vi "ConvertEventListToTriggerEvents.vi"(11 "Event List":string) -> (3 "Trigger Events":enum16{"Source", "Delay", "Sense", "None"}[](array[ring]))   [LabVIEW 2014, in "Keithley-6482-Visa.lvlib"]
uses:
  Keithley-6482-Visa.lvlib
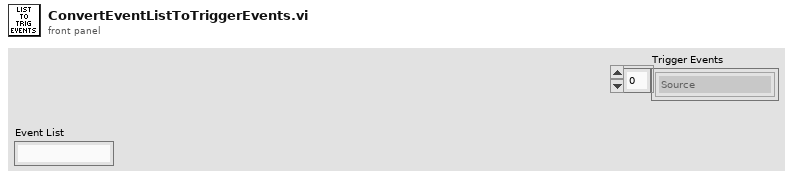
[diagram p1: front panel]
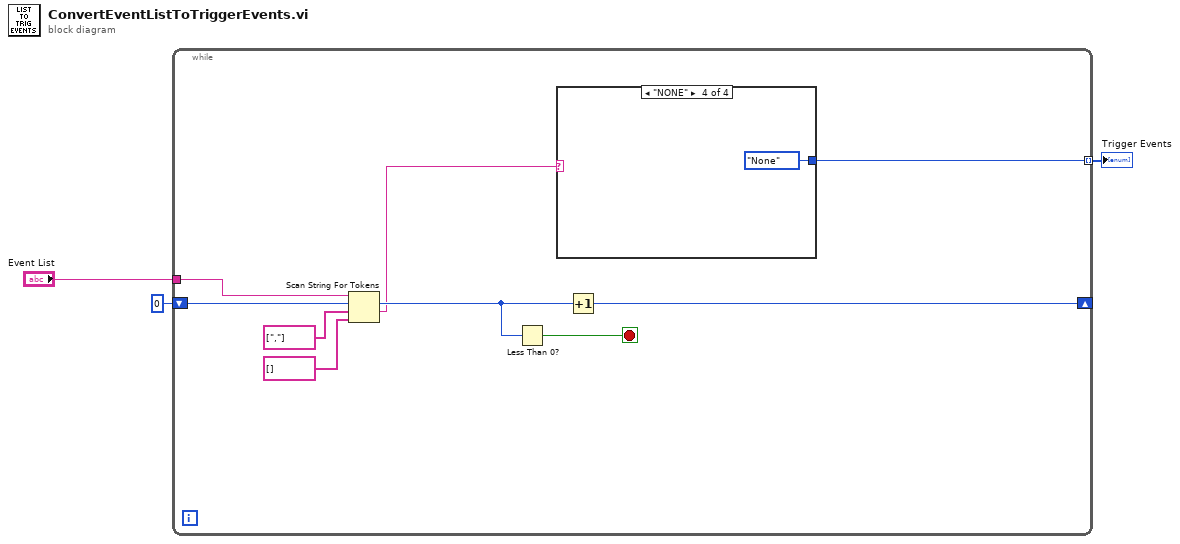
[diagram p0: block diagram]
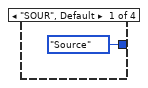
[diagram p2: hidden frame]
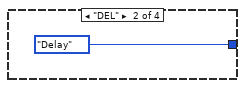
[diagram p3: hidden frame]
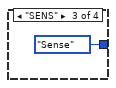
[diagram p4: hidden frame]
diagram:
  n1 = while {
    shift-right: [w6] -> _
    shift-left: 0 ("offset past token") -> [w12]
    tunnel: "Event List" -> [w9]
    tunnel: [w5] -> w1 mode=indexing
    stop <- w8 stop-if-true
    n2 = Scan String For Tokens(6:string[] [] ("delimiters (\\s,\\t,\\r,\\n)"), 7:string[] [","] ("delimiters (\\s,\\t,\\r,\\n)"), 8:w12, 9:w9) -> (1:w4:string, 2:w7:i32)  [unwired: 2 in, 2 out]
    n3 = Less Than 0?(x=w7) -> (x < 0?=w8:bool)
    n4 = case shown="\"NONE\"" w4 {
      tunnel: [enum16{"Source", "Delay", "Sense", "None"}."Source" ("Trigger Event") enum16{"Source", "Delay", "Sense", "None"}."Delay" ("Trigger Event") enum16{"Source", "Delay", "Sense", "None"}."Sense" ("Trigger Event") enum16{"Source", "Delay", "Sense", "None"}."None" ("Trigger Event")] -> w5
      frame "SOUR", Default {
      }
      frame "DEL" {
      }
      frame "SENS" {
      }
      frame "NONE" {
      }
    }
    n5 = Increment(x=w7) -> (x+1=w6:i32)
  }
  "Trigger Events" <- w1
